vi "IVCurveFit.vi"(11 "IVData":dbl[][](array[numeric])) -> (0 "error out":errorcluster, 1 "best fit parameters":dbl[](array[numeric]), 2 "Conductance":dbl, 3 "Capacitance":dbl)   [LabVIEW 2020]
uses:
  <vilib>/Analysis/6fits.llb/Curve Fitting Criteria.ctl
  <vilib>/gmath/NumericalOptimization/Nonlinear Curve Fit LM formula string.vi
  <vilib>/Analysis/NI_AALPro.lvlib
  <vilib>/gmath/NI_Gmath.lvlib
panel:
  out "XY Graph 2":cluster{"IVData":dbl[], "IVData":dbl[]}(graph)
  out "XY Graph":cluster{dbl[], dbl[]}[](graph)
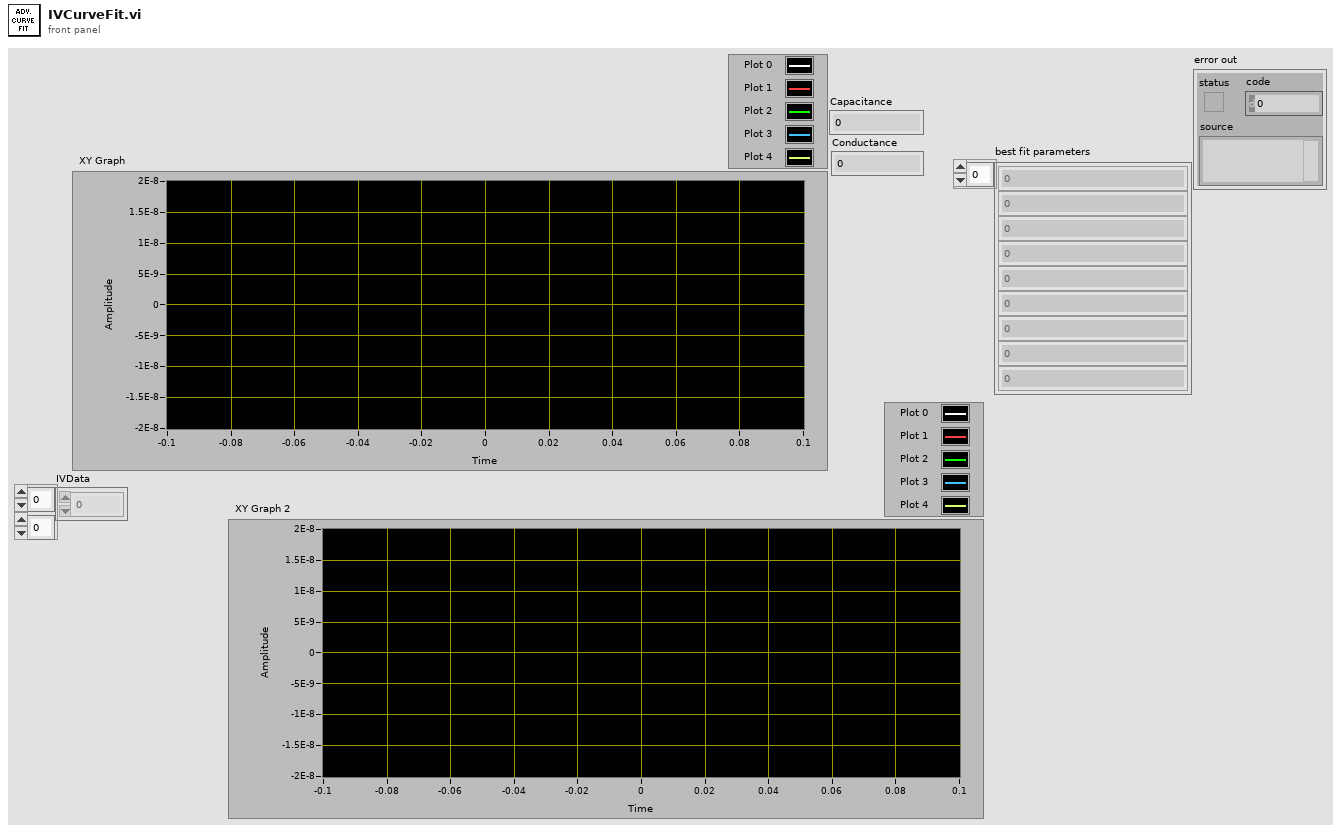
[diagram p1: front panel]
types:
  T1 = cluster{"model":string, "Parameters":string[], "x":string}
  T2 = typedef "NI_AALPro.lvlib/Curve Fitting Criteria.ctl" = u16
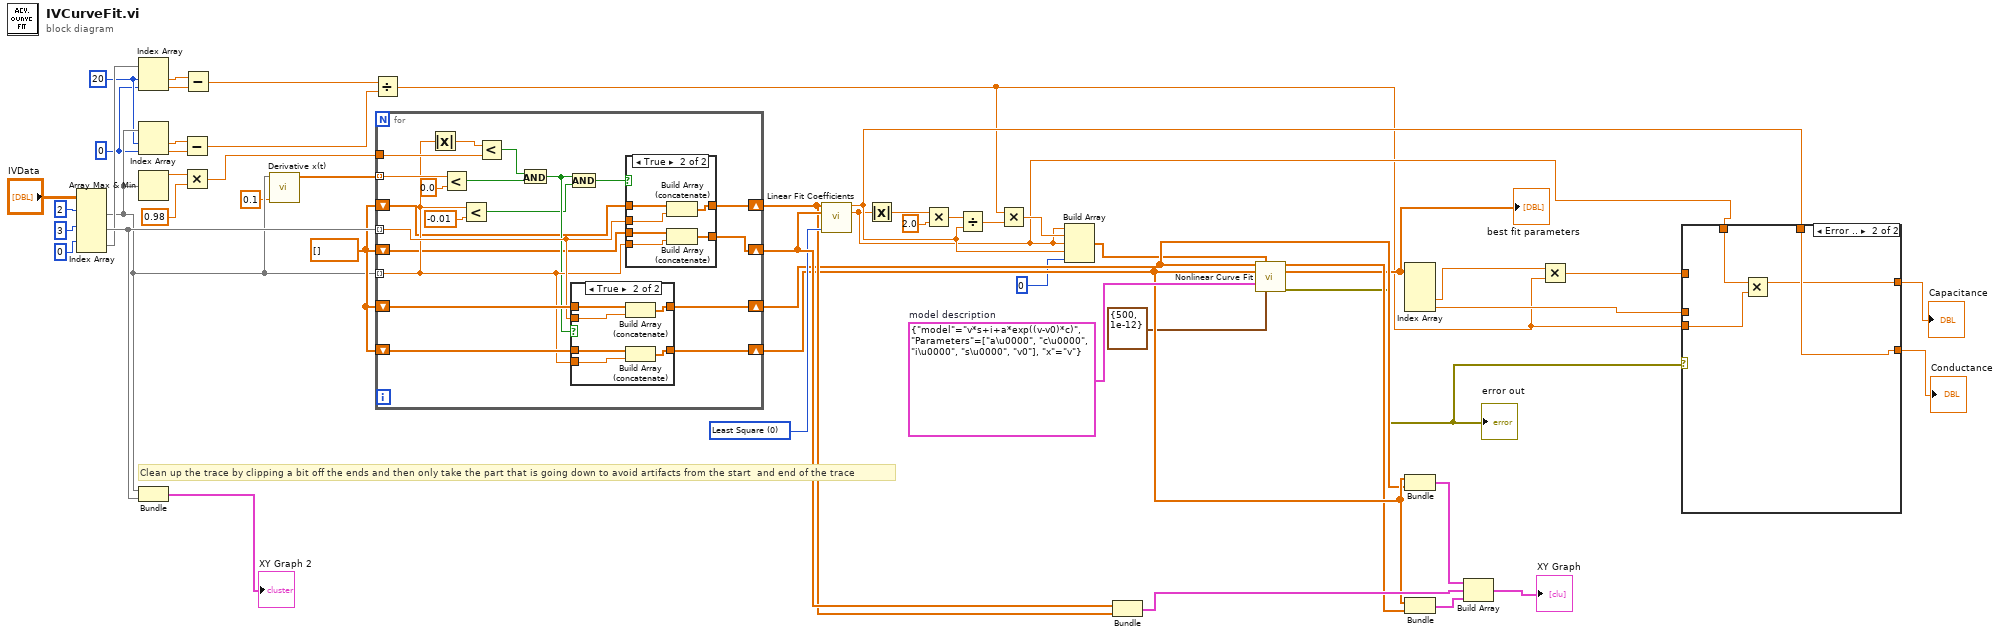
[diagram p0: block diagram]
diagram:
  w18 = 0 ("index")
  w19 = 20 ("index")
  w34 = T1 {"model"="v*s+i+a*exp((v-v0)*c)", "Parameters"=["a\u0000", "c\u0000", "i\u0000", "s\u0000", "v0"], "x"="v"}  # model description
  w40 = T2 0 items=["Least Square", "Least Absolute Residual", "Bisquare"] ("method")
  w43 = dbl[] []
  # "Clean up the trace by clipping a bit off the ends and then only take the part that is going down to avoid artifacts from the start  and end of the trace"
  n1 = Index Array(array="IVData", index (row) #1=2 ("index (row)"), index (row) #2=3 ("index (row)"), index (row) #3=0 ("index (row)")) -> (element #1=w20:dbl[], element #2=w46:dbl[], element #3=w23:dbl[])  [unwired: 3 in]
  n2 = Index Array(array=w23, index #1=w19, index #2=w18) -> (element #1=w22:dbl, element #2=w21:dbl)
  n3 = Index Array(array=w20, index #1=w19, index #2=w18) -> (element #1=w17:dbl, element #2=w16:dbl)
  n4 = Array Max & Min(array=w20) -> (max value=w51:dbl)  [unwired: 3 out]
  n5 = Bundle("IVData"=w20, "IVData"=w46) -> (→"XY Graph 2":cluster{"IVData":dbl[], "IVData":dbl[]})  [unwired: 1 in]
  n6 = Subtract(x=w17, y=w16) -> (x-y=w15:dbl)
  n7 = Multiply(x=w51, y=0.98) -> (x*y=w28:dbl)
  n8 = Subtract(x=w22, y=w21) -> (x-y=w14:dbl)
  n9 = call <vilib>:"Derivative x(t).vi"("dt"=0.1, "X"=w20) -> ("dX/dt"=w44:dbl[])  [unwired: 8 in, 1 out]
  n10 = Divide(x=w14, y=w15) -> (x/y=w1:dbl)
  n11 = for {
    tunnel: w28 -> [w68]
    tunnel: w20 -> [w59] mode=indexing
    tunnel: w46 -> [w60] mode=indexing
    shift-right: [w71] -> w33
    shift-left: w43 -> [w62]
    shift-right: [w70] -> w32
    shift-left: w43 -> [w61]
    tunnel: w44 -> [w66] mode=indexing
    shift-right: [w64] -> w41
    shift-left: w43 -> [w54]
    shift-right: [w63] -> w39
    shift-left: w43 -> [w53]
    n12 = Absolute Value(x=w59) -> (abs(x)=w69:dbl)
    n13 = Less?(x=w66, y=0.0) -> (x < y?=w52:bool)
    n14 = Less?(x=w59, y=-0.01) -> (x < y?=w56:bool)
    n15 = Less?(x=w69, y=w68) -> (x < y?=w67:bool)
    n16 = And(x=w67, y=w52) -> (x .and. y?=w57:bool)
    n17 = And(x=w57, y=w56) -> (x .and. y?=w55:bool)
    n18 = case shown="True" w57 {
      tunnel: w62 -> [w81 w87]
      tunnel: w61 -> [w80 w86]
      tunnel: [w81 w85] -> w71
      tunnel: [w80 w84] -> w70
      tunnel: w59 -> [_ w83]
      tunnel: w60 -> [_ w82]
      frame False {
      }
      frame True {
        n19 = Build Array (concatenate)(w86, w82) -> (w84:dbl[])
        n20 = Build Array (concatenate)(w87, w83) -> (w85:dbl[])
      }
    }
    n21 = case shown="True" w55 {
      tunnel: w54 -> [w73 w79]
      tunnel: w53 -> [w72 w78]
      tunnel: [w73 w77] -> w64
      tunnel: [w72 w76] -> w63
      tunnel: w59 -> [_ w75]
      tunnel: w60 -> [_ w74]
      frame False {
      }
      frame True {
        n22 = Build Array (concatenate)(w78, w74) -> (w76:dbl[])
        n23 = Build Array (concatenate)(w79, w75) -> (w77:dbl[])
      }
    }
  }
  n24 = call <vilib>:"Linear Fit Coefficients.vi"("Y"=w39, "X"=w41, "method"=w40) -> ("slope"=w3:dbl, "intercept"=w2:dbl)  [unwired: 10 in, 1 out]
  n25 = Absolute Value(x=w2) -> (abs(x)=w38:dbl)
  n26 = Multiply(x=w38, y=2.0) -> (x*y=w36:dbl)
  n27 = Divide(x=w36, y=w3) -> (x/y=w35:dbl)
  n28 = Multiply(x=w1, y=w35) -> (x*y=w4:dbl)
  n29 = Build Array(w2, w4, w2, w3, 0) -> (w29:dbl[])
  n30 = Bundle(w41, w39) -> (w42:cluster{dbl[], dbl[]})  [unwired: 1 in]
  n31 = call-poly <vilib>:"Nonlinear Curve Fit.vi"("Y"=w32, "initial parameters"=w29, "X"=w33, "model description"=w34, "termination"=cluster{"max iteration":i32, "tolerance":dbl} {"max iteration"=500, "tolerance"=1e-12}) -> ("best nonlinear fit"=w31:dbl[], "best fit parameters"=w13:dbl[], "error out"=w9:errorcluster)  [unwired: 6 in, 2 out]
  "best fit parameters" <- w13
  "error out" <- w9
  n32 = Index Array(array=w13) -> (element #3=w12:dbl, element #4=w8:dbl)  [unwired: 4 in, 2 out]
  n33 = Bundle(w33, w32) -> (w45:cluster{dbl[], dbl[]})  [unwired: 1 in]
  n34 = Bundle(w33, "best nonlinear fit"=w31) -> (w30:cluster{dbl[], "best nonlinear fit":dbl[]})  [unwired: 1 in]
  n35 = Build Array(w45, w42, w30) -> (→"XY Graph":cluster{dbl[], "best nonlinear fit":dbl[]}[])
  n36 = Multiply(x=w12, y=w1) -> (x*y=w5:dbl)
  n37 = case shown="Error .." w9 {
    tunnel: [w89 w93] -> w7
    tunnel: w8 -> [w89 _]
    tunnel: [w88 w91] -> w6
    tunnel: w5 -> [w88 _]
    tunnel: w3 -> [_ w93]
    tunnel: w2 -> [_ w92]
    tunnel: w1 -> [_ w90]
    frame No Error {
    }
    frame Error {
      n38 = Multiply(x=w92, y=w90) -> (x*y=w91:dbl)
    }
  }
  "Capacitance" <- w6
  "Conductance" <- w7
